vi "AgilentMeasureTest.vi"() -> ()   [LabVIEW 2009]
uses:
  AgilentControl.ctl
  Channel Config.ctl
  <vilib>/Utility/file.llb/Write To Spreadsheet File (DBL).vi
  <instrlib>/Agilent 6000 Series/Agilent 6000 Series.lvlib
panel:
  in  "Plot Graph":bool
  out "Time per acq (ms)":dbl
  out "Elapsed Time (ms)":u32
  in  "Max Points":i32
  in  "Target File Path":path
  out "Close Error":errorcluster
  out "Waveform Chart":dbl[](graph)
  out "Loop Num":i32
  out "Measure Output":dbl[][](array[numeric])
  in  "stop":bool
  in  "Measurement Function (7: Frequency)":u16(ring)=7 items=["Amplitude", "Voltage Average", "Base", "Counter", "Delay", "Duty Cycle", "Fall Time", "Frequency", "Voltage Max", "Voltage Min", "Overshoot", "Voltage Vpp", "Period", "Phase", "Preshoot", "Rise Time", "Voltage RMS", "Top", "Width Positive", "X at Max Y", "X at Min Y"]
  out "Agilent Control Out":T1={"Trig?"=FALSE, "VISA session"="", "Setup to Load"="CH1", "Timeout (ms)"=10000, "Desired Samp"=enum."100", "Captured Samp"=0, "Desired Channels"=[]}
  in  "Agilent Control In":T1={"Trig?"=FALSE, "VISA session"="", "Setup to Load"="CH1", "Timeout (ms)"=10000, "Desired Samp"=enum."100", "Captured Samp"=0, "Desired Channels"=[]}
  out "Data Download Error":errorcluster[](array[cluster])
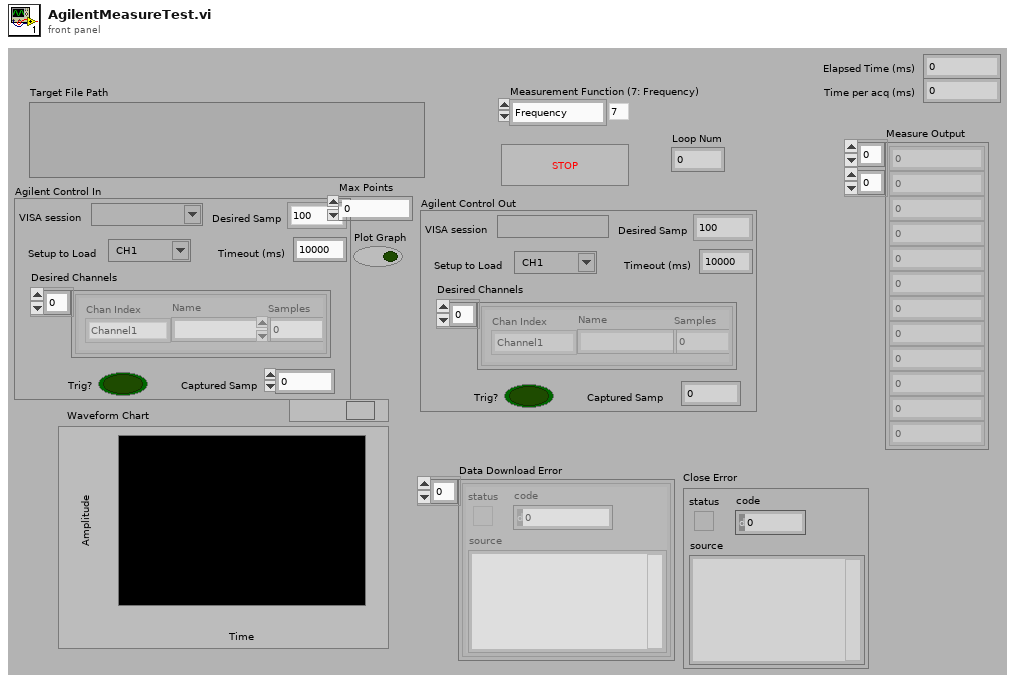
[diagram p1: front panel]
types:
  T1 = typedef "AgilentControl.ctl" = cluster{"Trig?":bool, "VISA session":refnum<visa-resource-name>, "Setup to Load":string, "Timeout (ms)":u32, "Desired Samp":enum32{"100", "250", "500", "1000", "2000", "5000", "10000", "20000", "50000", "100000", "200000", "500000", "1000000", "2000000", "4000000", "8000000"}, "Captured Samp":i32, "Desired Channels":T2[]}
  T2 = typedef "Channel Config.ctl" = cluster{"Chan Index":enum16{"Channel1", "Channel2", "Channel3", "Channel4", "MATH"}, "Name":string, "Samples":i32}
  T3 = enum16{"Channel1", "Channel2", "Channel3", "Channel4", "MATH"}
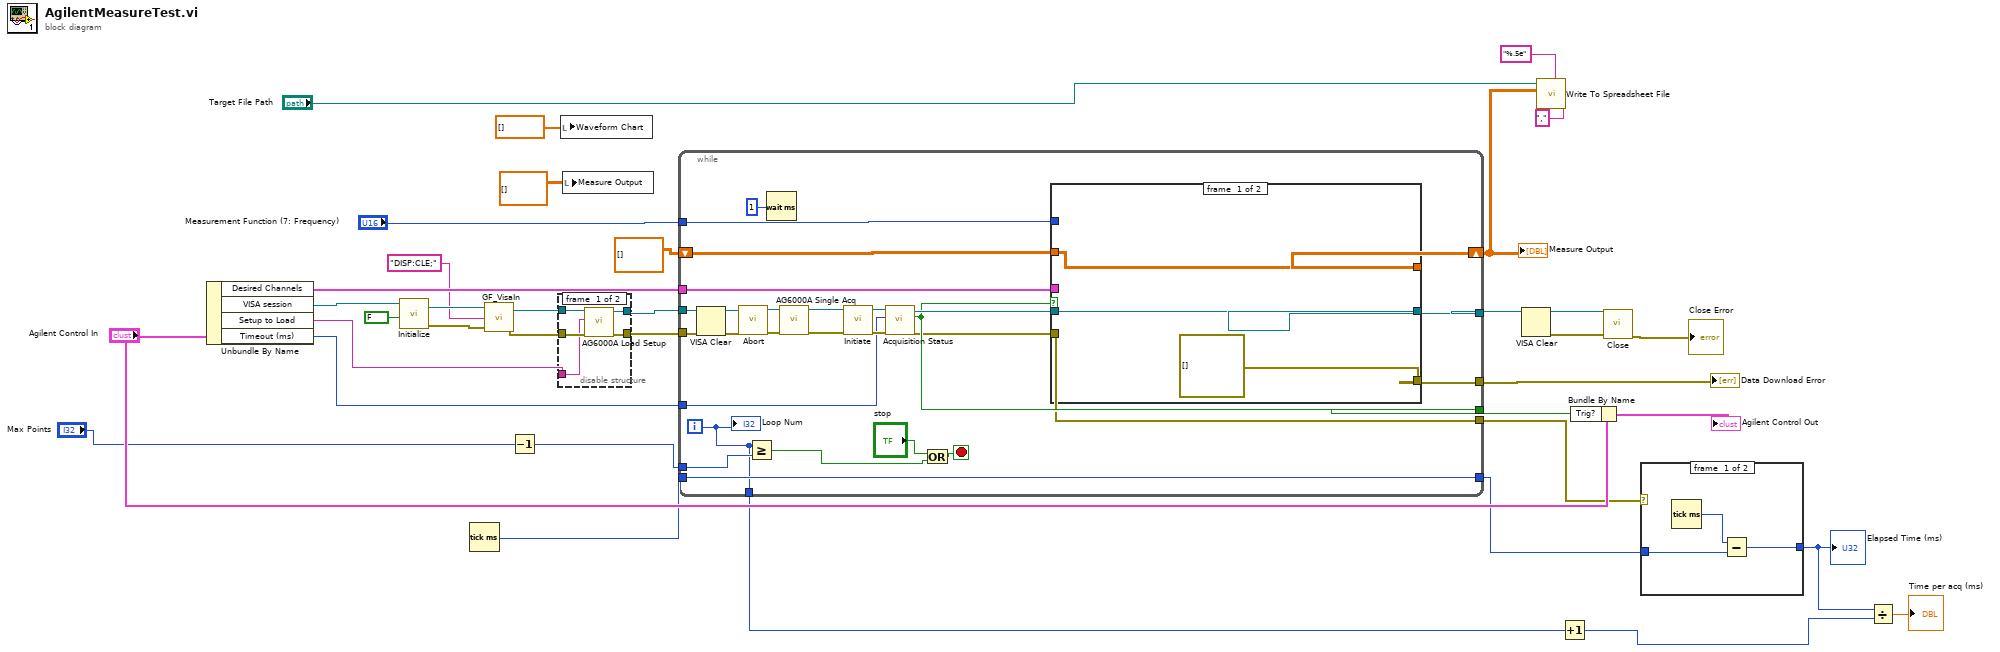
[diagram p0: block diagram]
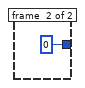
[diagram p2: hidden frame]
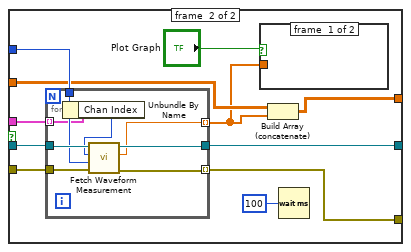
[diagram p3: hidden frame]
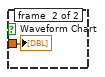
[diagram p4: hidden frame]
diagram:
  n1 = Unbundle By Name("Agilent Control In") -> ("Desired Channels"=w36:T2[], "VISA session"=w35:refnum<visa-resource-name>, "Setup to Load"=w33:string, "Timeout (ms)"=w32:u32)
  n2 = call <instrlib>:"Initialize.vi"("Reset? (T: Yes)"=FALSE, "VISA resource name"=w35) -> ("error out"=w17:errorcluster, "VISA resource name out"=w18:refnum<visa-resource-name>)  [unwired: 8 in]
  n3 = Tick Count (ms)() -> (millisecond timer value=w7:u32)
  n4 = call "GF_VisaIn.vi"("error in (no error)"=w17, "String"="DISP:CLE;", "VISA resource name"=w18) -> ("error out"=w16:errorcluster, "VISA resource name out"=w15:refnum<visa-resource-name>)
  n5 = Decrement(x="Max Points") -> (x-1=w9:i32)
  n6 = disable-structure shown="Enabled" {
    disable-tunnel: [w42 w43] -> w27
    disable-tunnel: [w41 w44] -> w26
    disable-tunnel: w15 -> [w40 w43]
    disable-tunnel: w16 -> [w39 w44]
    disable-tunnel: w33 -> [w38 _]
    frame #0 {
      n7 = call "AG6000A Load Setup.vi"("error in (no error)"=w39, "Setup to Load"=w38, "VISA session"=w40) -> ("error out"=w41:errorcluster, "dup VISA session"=w42:refnum<visa-resource-name>)  [unwired: 7 in]
    }
    frame #1 {
    }
  }
  n8 = local write "Waveform Chart"(dbl[] [] ("Waveform Chart")) -> ()
  n9 = local write "Measure Output"(dbl[][] [] ("Measure Output")) -> ()
  n10 = while {
    tunnel: [w58] -> w21
    tunnel: [w70] -> w37
    tunnel: w36 -> [w67]
    tunnel: w32 -> [w66]
    tunnel: [w65] -> w30
    tunnel: "Measurement Function (7: Frequency)" -> [w64]
    tunnel: w27 -> [w56]
    tunnel: w26 -> [w53]
    shift-right: [w60] -> w10
    shift-left: dbl[][] [] -> [w61]
    tunnel: [w57] -> w6
    tunnel: w9 -> [w50]
    tunnel: w7 -> [w48]
    tunnel: [w48] -> w5
    tunnel: [w47] -> w2
    i -> [w47]
    stop <- w51 stop-if-true
    n11 = VISA Clear(VISA resource name=w56, error in (no error)=w53) -> (VISA resource name out=w55:refnum<visa-resource-name>, error out=w54:errorcluster)
    n12 = call <instrlib>:"Abort.vi"("error in (no error)"=w54, "VISA resource name"=w55) -> ("error out"=w45:errorcluster, "VISA resource name out"=w46:refnum<visa-resource-name>)  [unwired: 8 in]
    n13 = Greater Or Equal?(x=w47, y=w50) -> (x >= y?=w49:bool)
    n14 = Wait (ms)(milliseconds to wait=u32 1) -> ()  [unwired: 1 out]
    n15 = call "AG6000A Single Acq.vi"("error in (no error)"=w45, "VISA session"=w46) -> ("error out"=w62:errorcluster, "dup VISA session"=w63:refnum<visa-resource-name>)  [unwired: 8 in]
    n16 = call <instrlib>:"Initiate.vi"("error in (no error)"=w62, "VISA resource name"=w63) -> ("error out"=w68:errorcluster, "VISA resource name out"=w69:refnum<visa-resource-name>)  [unwired: 8 in]
    n17 = call <instrlib>:"Acquisition Status.vi"("error in (no error)"=w68, "Timeout (10000 ms)"=w66, "VISA resource name"=w69) -> ("error out"=w57:errorcluster, "Acquisition Complete?"=w65:bool, "VISA resource name out"=w71:refnum<visa-resource-name>)  [unwired: 6 in]
    n18 = Or(x="stop", y=w49) -> (x .or. y?=w51:bool)
    n19 = case shown="True" w65 {
      tunnel: w71 -> [w72 w85]
      tunnel: w57 -> [_ w84]
      tunnel: w67 -> [_ w83]
      tunnel: [w72 w82] -> w58
      tunnel: [errorcluster[] [] w81] -> w70
      tunnel: w64 -> [_ w80]
      tunnel: w61 -> [w73 w79]
      tunnel: [w73 w78] -> w60
      frame #0 {
      }
      frame #1 {
        n20 = for {
          tunnel: w85 -> [w94]
          tunnel: w84 -> [w93]
          tunnel: w83 -> [w88] mode=indexing
          tunnel: [w91] -> w82
          tunnel: [w90] -> w81 mode=indexing
          tunnel: w80 -> [w92]
          tunnel: [w89] -> w77 mode=indexing
          n21 = Unbundle By Name(w88) -> ("Chan Index"=w87:T3)
          n22 = call <instrlib>:"Fetch Waveform Measurement.vi"("error in (no error)"=w93, "Measurement Function (7: Frequency)"=w92, "Source 1 (0: Channel 1)"=w87, "VISA resource name"=w94) -> ("error out"=w90:errorcluster, "Measured Value"=w89:dbl, "VISA resource name out"=w91:refnum<visa-resource-name>)  [unwired: 5 in]
        }
        n23 = case shown="True" "Plot Graph" {
          tunnel: w77 -> [_ w86]
          frame #0 {
          }
          frame #1 {
            "Waveform Chart" <- w86
          }
        }
        n24 = Build Array (concatenate)(w79, w77) -> (w78:dbl[][])
        n25 = Wait (ms)(milliseconds to wait=u32 100) -> ()  [unwired: 1 out]
      }
    }
    "Loop Num" <- w47
  }
  "Data Download Error" <- w37
  "Measure Output" <- w10
  n26 = VISA Clear(VISA resource name=w21) -> (VISA resource name out=w20:refnum<visa-resource-name>, error out=w19:errorcluster)  [unwired: 1 in]
  n27 = call-poly <vilib>:"Write To Spreadsheet File.vi"("delimiter (\\t)"="," ("delimiter (\\t)"), "format (%.3f)"="%.5e", "2D data"=w10, "file path (dialog if empty)"="Target File Path") -> ()  [unwired: 4 in, 1 out]
  n28 = Increment(x=w2) -> (x+1=w3:i32)
  n29 = Bundle By Name(cluster="Agilent Control In", "Trig?"=w30) -> (→"Agilent Control Out":T1)
  n30 = call <instrlib>:"Close.vi"("error in (no error)"=w19, "VISA resource name"=w20) -> ("error out"=→"Close Error":errorcluster)  [unwired: 9 in]
  n31 = case shown="No Error" w6 {
    tunnel: w5 -> [w96 _]
    tunnel: [w95 u32 0] -> w4
    frame #0 {
      n32 = Tick Count (ms)() -> (millisecond timer value=w97:u32)
      n33 = Subtract(x=w97, y=w96) -> (x-y=w95:u32)
    }
    frame #1 {
    }
  }
  "Elapsed Time (ms)" <- w4
  n34 = Divide(x=w4, y=w3) -> (x/y=→"Time per acq (ms)":dbl)
